vi "PPMS field set point.vi"(0 "GPIB address":string="15", 1 "error in (no error)":errorcluster) -> (2 "Field set point (Oe)":dbl format="%.2f", 3 "Set rate (Oe/s)":dbl format="%.2f", 4 "Magnet Mode":string, 5 "error out":errorcluster)   [LabVIEW 2018]
doc: "This VI returns the set point of the magnetic field, the rate of change of the field, and the mode that the magnet is in. Note that this is not the actual strength of the field, just the point towards which it is changing."
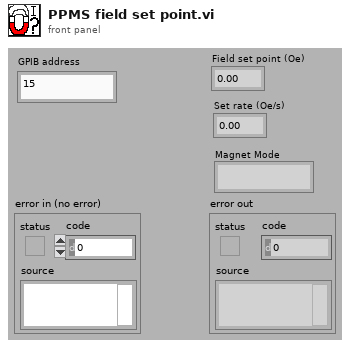
[diagram p1: front panel]
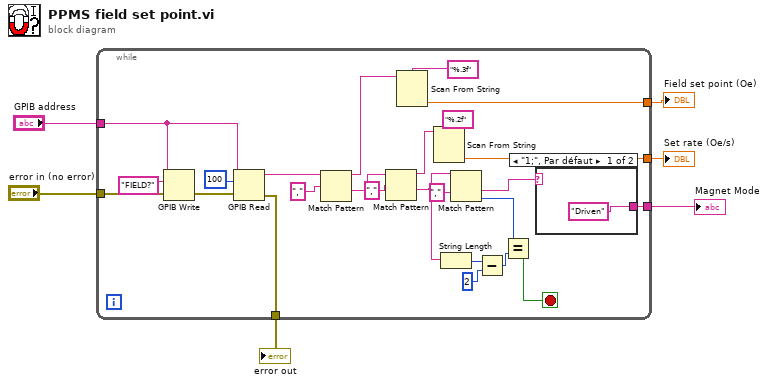
[diagram p0: block diagram]
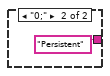
[diagram p2: hidden frame]
diagram:
  n1 = while {
    tunnel: "GPIB address" -> [w31]
    tunnel: "error in (no error)" -> [w30]
    tunnel: [w28] -> w4
    tunnel: [w23] -> w3
    tunnel: [w18] -> w2
    tunnel: [w7] -> w1
    stop <- w13 stop-if-true
    n2 = GPIB Write(0:w31, 1:"FIELD?", 3:w30) -> (6:w29:errorcluster)  [unwired: 3 out]
    n3 = GPIB Read(0:w31, 1:100, 3:w29) -> (5:w25:string, 7:w28:errorcluster)  [unwired: 3 out]
    n4 = Match Pattern(string=w25, regular expression=",") -> (before substring=w20:string, after substring=w12:string)  [unwired: 3 out]
    n5 = Match Pattern(string=w12, regular expression=",") -> (before substring=w19:string, after substring=w11:string)  [unwired: 3 out]
    n6 = Scan From String(format string="%.3f", input string=w20) -> (output 1=w23:dbl)  [unwired: 2 in, 4 out]
    n7 = Scan From String(format string="%.2f", input string=w19) -> (output 1=w18:dbl)  [unwired: 2 in, 4 out]
    n8 = String Length(string=w11) -> (length=w15:i32)
    n9 = Match Pattern(string=w11, regular expression=",") -> (after substring=w8:string, offset past match=w9:i32)  [unwired: 3 out]
    n10 = Subtract(x=w15, y=2) -> (x-y=w16:i32)
    n11 = Equal?(x=w9, y=w16) -> (x = y?=w13:bool)
    n12 = case shown="\"1;\", Par défaut" w8 {
      tunnel: ["Driven" "Persistent"] -> w7
      frame "1;", Default {
      }
      frame "0;" {
      }
    }
  }
  "error out" <- w4
  "Field set point (Oe)" <- w3
  "Set rate (Oe/s)" <- w2
  "Magnet Mode" <- w1
